vi "Logo Exaprom.vi"(0 "PDFStamper GetOverContent":refnum<k24>, 1 "text1":string="Exaprom inc.", 3 "Text2":string="Consultation et essais en génie des\nmatériaux et en énergies durables", 9 "Facteur":sgl=0.2, 11 "error in (no error)":errorcluster, 13 "Page dimensions":T1={"Start at page"=1, "Orientation"=enum."Portrait", "widht"=612.0, "height"=792.0, "Margin left"=72.0, "Margin right"=72.0, "Margin top"=72.0, "Margin bottom"=72.0}) -> (4 "PDFStamper GetOverContent duplicate":refnum<k24>, 15 "error out":errorcluster)   [LabVIEW 2013]
doc: "Version 1.0\nDeveloped by Jean-Marc Simard\nCopyright © 2010, Exaprom Inc.\nAll rights reserved.\nLicense: BSD\n\nWith iTextSharp Library\n(http://itextsharp.sourceforge.net)"
uses:
  C:/Users/MaxCorp/Documents/GitHub/TopView/DLL/itextsharp.dll
  DLL/itextsharp.dll
  Controls/Header footer horiz alignment.ctl
  Controls/Font size.ctl
  Controls/Font color.ctl
  Controls/Font cluster.ctl
  Controls/Cell Vertical alignment.ctl
  Controls/Page Orientation.ctl
  Controls/Page dimensions.ctl
panel:
  in  "Alignment":T3
  in  "Vertical Alignement":T4=enum."BOTTOM"
  # "Consultation et essais en génie des\nmatériaux et en énergies durables"
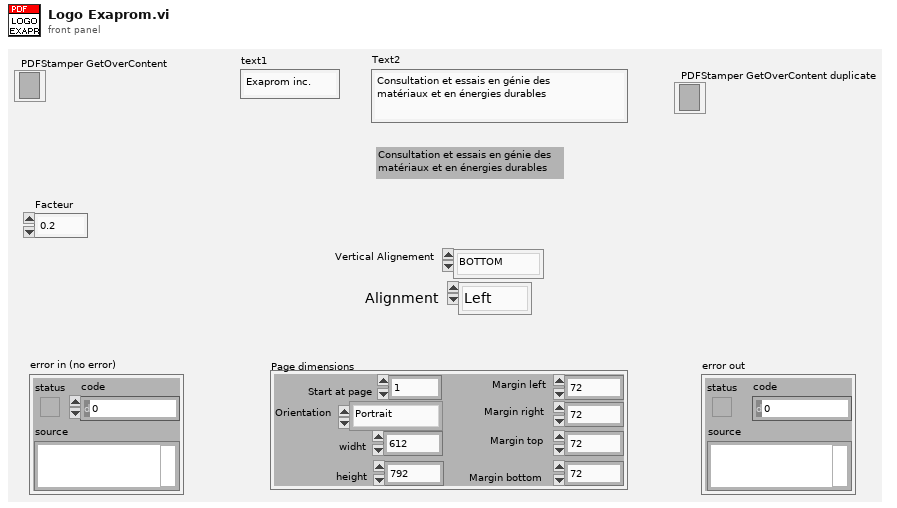
[diagram p1: front panel]
types:
  T1 = typedef "Page dimensions.ctl" = cluster{"Start at page":i32, "Orientation":T2, "widht":sgl, "height":sgl, "Margin left":sgl, "Margin right":sgl, "Margin top":sgl, "Margin bottom":sgl}
  T2 = typedef "Page Orientation.ctl" = enum16{"Portrait", "Landscape"}
  T3 = typedef "Header footer horiz alignment.ctl" = enum16{"Left", "Center", "Right"}
  T4 = typedef "Cell Vertical alignment.ctl" = enum16{"TOP", "MIDDLE", "BOTTOM"}
  T5 = typedef "Font size.ctl" = sgl
  T6 = typedef "Font cluster.ctl" = cluster{"Name":string, "Size":T5, "Color":T7, "Style":cluster{"Bold":bool, "Italic":bool, "Underline":bool, "Strikeout":bool}}
  T7 = typedef "Font color.ctl" = u32
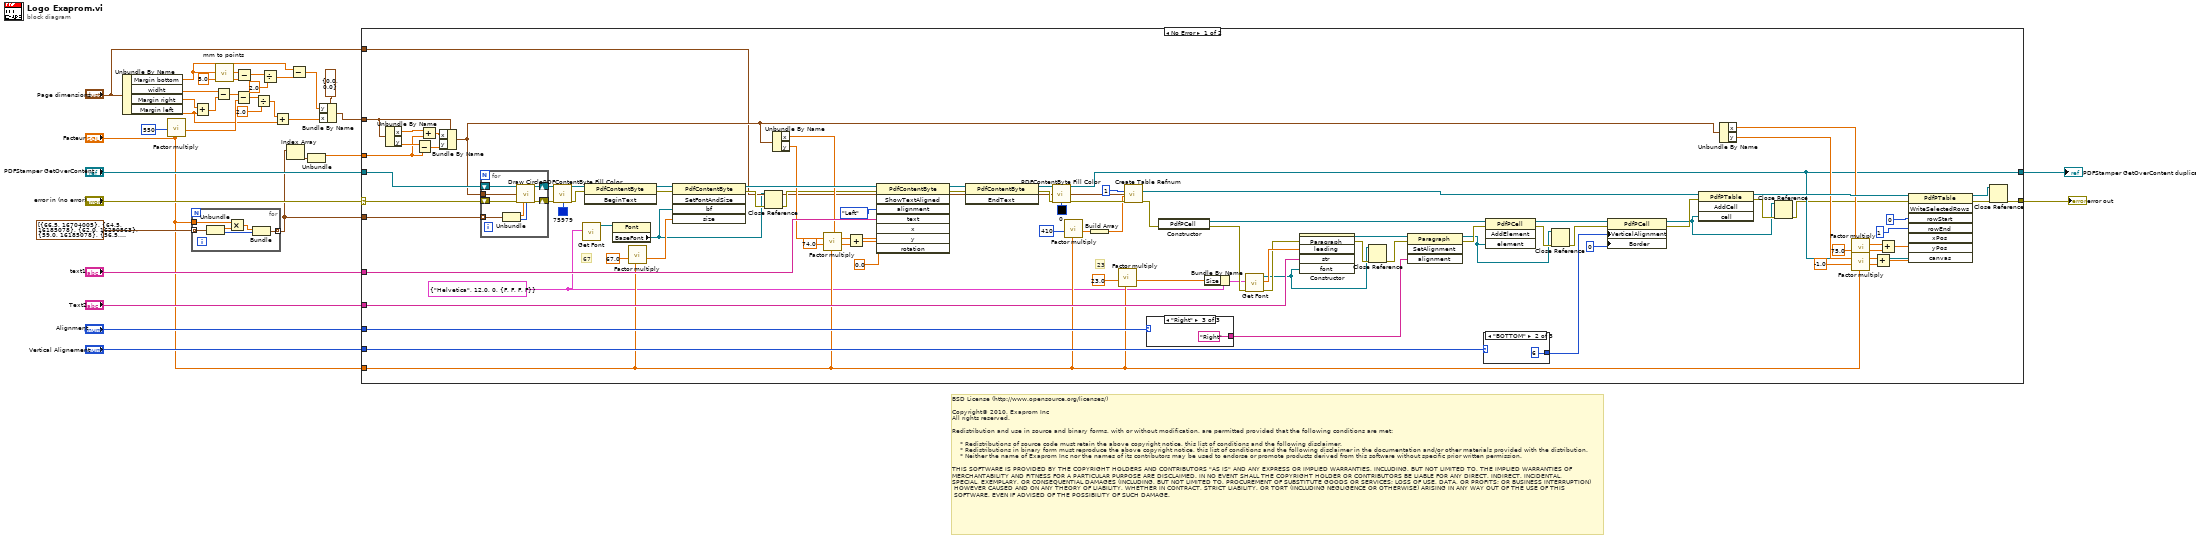
[diagram p0: block diagram]
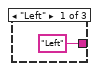
[diagram p2: hidden frame]
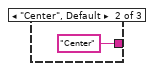
[diagram p3: hidden frame]
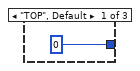
[diagram p4: hidden frame]
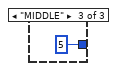
[diagram p5: hidden frame]
diagram:
  # "BSD License (http://www.opensource.org/licenses/)\n\nCopyright© 2010, Exaprom Inc\nAll rights reserved.\n\nRedistribution and use in source and binary forms, with or without modification, are permitted provided that the following conditions are met:\n\n    * Redistributions of source code must retain the above copyright notice, this list of conditions and the following disclaimer.\n    * Redistributions in binary form must reproduce the above copyright notice, this list of conditions and the following disclaimer in the documentation and/or other materials provided with the distribution.\n    * Neither the name of Exaprom Inc nor the names of its contributors may be used to endorse or promote products derived from this software without specific prior written permission.\n\nTHIS SOFTWARE IS PROVIDED BY THE COPYRIGHT HOLDERS AND CONTRIBUTORS \"AS IS\" AND ANY EXPRESS OR IMPLIED WARRANTIES, INCLUDING, BUT NOT LIMITED TO, THE IMPLIED WARRANTIES OF \nMERCHANTABILITY AND FITNESS FOR A PARTICULAR PURPOSE ARE DISCLAIMED. IN NO EVENT SHALL THE COPYRIGHT HOLDER OR CONTRIBUTORS BE LIABLE FOR ANY DIRECT, INDIRECT, INCIDENTAL,\nSPECIAL, EXEMPLARY, OR CONSEQUENTIAL DAMAGES (INCLUDING, BUT NOT LIMITED TO, PROCUREMENT OF SUBSTITUTE GOODS OR SERVICES; LOSS OF USE, DATA, OR PROFITS; OR BUSINESS INTERRUPTION)\n HOWEVER CAUSED AND ON ANY THEORY OF LIABILITY, WHETHER IN CONTRACT, STRICT LIABILITY, OR TORT (INCLUDING NEGLIGENCE OR OTHERWISE) ARISING IN ANY WAY OUT OF THE USE OF THIS\n SOFTWARE, EVEN IF ADVISED OF THE POSSIBILITY OF SUCH DAMAGE."
  n1 = Unbundle By Name("Page dimensions") -> ("Margin bottom"=w4:sgl, "widht"=w27:sgl, "Margin right"=w26:sgl, "Margin left"=w20:sgl)
  n2 = call "Factor multiply.vi"("factor"="Facteur", "Numeric IN"=550) -> ("Numeric OUT"=w23:sgl)  [unwired: 6 out]
  n3 = for {
    tunnel: cluster{"r":sgl, "Color":u32}[] [{"r"=66.5, "Color"=16704005}, {"r"=64.5, "Color"=16185078}, {"r"=62.0, "Color"=16290563}, {"r"=59.0, "Color"=16185078}, {"r"=56.5, "Color"=16290563}, {"r"=52.5, "Color"=16185078}, {"r"=50.0, "Color"=16711680}] -> [w40] mode=indexing
    tunnel: "Facteur" -> [w38]
    tunnel: [w35] -> w12 mode=indexing
    n4 = Unbundle(w40) -> ("r"=w39:sgl, "Color"=w36:u32)
    n5 = Multiply(x=w38, y=w39) -> (x*y=w37:sgl)
    n6 = Bundle(w37, "Color"=w36) -> (w35:cluster{sgl, "Color":u32})  [unwired: 1 out]
  }
  n7 = Add(x=w26, y=w20) -> (x+y=w25:sgl)
  n8 = Subtract(x=w27, y=w25) -> (x-y=w24:sgl)
  n9 = call "mm to points.vi"("mm"=sgl 5.0) -> ("points"=w10:sgl)  [unwired: 4 out]
  n10 = Subtract(x=w24, y=w23) -> (x-y=w22:sgl)
  n11 = Subtract(x=w4, y=w10) -> (x-y=w6:sgl)
  n12 = Divide(x=w22, y=2.0) -> (x/y=w8:dbl)
  n13 = Divide(x=w6, y=2.0) -> (x/y=w5:dbl)
  n14 = Add(x=w8, y=w20) -> (x+y=w19:dbl)
  n15 = Index Array(array=w12) -> (element=w13:cluster{sgl, "Color":u32})  [unwired: 1 in]
  n16 = Subtract(x=w4, y=w5) -> (x-y=w2:dbl)
  n17 = Unbundle(w13) -> (w11:sgl)  [unwired: 1 out]
  n18 = Bundle By Name(cluster=cluster{"x":sgl, "y":sgl} {"x"=0.0, "y"=0.0} ("Position"), "y"=w2, "x"=w19) -> (w18:cluster{"x":sgl, "y":sgl})
  n19 = case shown="No Error" "error in (no error)" {
    selector: "error in (no error)" -> [w61 w144]
    tunnel: [w96 w144] -> w33
    tunnel: w18 -> [w67 _]
    tunnel: "Facteur" -> [w60 _]
    tunnel: "text1" -> [w92 _]
    tunnel: "Text2" -> [w88 _]
    tunnel: "Alignment" -> [w87 _]
    tunnel: "Vertical Alignement" -> [w86 _]
    tunnel: "PDFStamper GetOverContent" -> [w62 w143]
    tunnel: [w65 w143] -> w16
    tunnel: w12 -> [w58 _]
    tunnel: w11 -> [w57 _]
    tunnel: "Page dimensions" -> [w44 _]
    frame No Error {
      w42 = T6 {"Name"="Helvetica", "Size"=12.0, "Color"=0, "Style"={"Bold"=FALSE, "Italic"=FALSE, "Underline"=FALSE, "Strikeout"=FALSE}} ("Font")
      # "23"
      # "67"
      n20 = Unbundle By Name(w67) -> ("x"=w71:sgl, "y"=w70:sgl)
      n21 = Subtract(x=w70, y=w57) -> (x-y=w68:sgl)
      n22 = Add(x=w71, y=w57) -> (x+y=w69:sgl)
      n23 = Bundle By Name(cluster=w67, "x"=w69, "y"=w68) -> (w59:cluster{"x":sgl, "y":sgl})
      n24 = for {
        tunnel: w58 -> [w136] mode=indexing
        shift-right: [w133] -> w64
        shift-left: w62 -> [w134]
        shift-right: [w132] -> w63
        shift-left: w61 -> [w131]
        tunnel: w59 -> [w130]
        n25 = Unbundle(w136) -> (w129:sgl, "Color"=w135:u32)
        n26 = call "Draw Circle.vi"("GetOverContent IN"=w134, "Center"=w130, "error in (no error)"=w131, "r"=w129, "Color Box"=w135) -> ("GetOverContent OUT"=w133:refnum<k24>, "error out"=w132:errorcluster)  [unwired: 1 in, 8 out]
      }
      n27 = call "PDFContentByte Fill Color.vi"("PDFContentByte"=w64, "error in (no error)"=w63, "Color Box"=u32 75979) -> ("PDFContentByte duplicate"=w45:refnum<k24>, "error out"=w124:errorcluster)  [unwired: 1 in, 10 out]
      n28 = call "Get Font.vi"("Font IN"=w42) -> ("Font"=w43:refnum<k24>)  [unwired: 7 in, 3 out]
      n29 = invoke class="PdfContentByte" method="BeginText"(reference=w45, error in=w124) -> (reference out=w117:refnum<k24>, error out=w122:errorcluster)  [unwired: 1 in, 1 out]
      n30 = property class="Font"(reference=w43) -> ("BaseFont"=w41:refnum<k24>)  [unwired: 1 in, 2 out]
      n31 = call "Factor multiply.vi"("factor"=w60, "Numeric IN"=sgl 67.0 ("size")) -> ("Numeric OUT"=w115:sgl)  [unwired: 6 out]
      n32 = invoke class="PdfContentByte" method="SetFontAndSize"(reference=w117, error in=w122, "bf"=w41, "size"=w115) -> (reference out=w121:refnum<k24>, error out=w56:errorcluster)  [unwired: 1 in, 3 out]
      n33 = Close Reference(reference=w41, error in (no error)=w56) -> (error out=w55:errorcluster)
      n34 = Unbundle By Name(w59) -> ("x"=w84:sgl, "y"=w85:sgl)
      n35 = call "Factor multiply.vi"("factor"=w60, "Numeric IN"=sgl 74.0 ("y")) -> ("Numeric OUT"=w82:sgl)  [unwired: 6 out]
      n36 = Add(x=w84, y=w82) -> (x+y=w81:sgl)
      n37 = invoke class="PdfContentByte" method="ShowTextAligned"(reference=w121, error in=w55, "alignment"=Header_footer_horiz_alignment."Left" ("Alignment 2"), "text"=w92, "x"=w81, "y"=w85, "rotation"=sgl 0.0) -> (reference out=w119:refnum<k24>, error out=w123:errorcluster)  [unwired: 1 in, 6 out]
      n38 = invoke class="PdfContentByte" method="EndText"(reference=w119, error in=w123) -> (reference out=w126:refnum<k24>, error out=w127:errorcluster)  [unwired: 1 in, 1 out]
      n39 = call "PDFContentByte Fill Color.vi"("PDFContentByte"=w126, "error in (no error)"=w127, "Color Box"=u32 0) -> ("PDFContentByte duplicate"=w65:refnum<k24>, "error out"=w97:errorcluster)  [unwired: 1 in, 10 out]
      n40 = call "Factor multiply.vi"("factor"=w60, "Numeric IN"=410) -> ("Numeric OUT"=w94:sgl)  [unwired: 6 out]
      n41 = Build Array(w94) -> (w93:sgl[])
      n42 = call "Factor multiply.vi"("factor"=w60, "Numeric IN"=T5 23.0 ("Size")) -> ("Numeric OUT"=w90:sgl)  [unwired: 6 out]
      n43 = call "Create Table Refnum.vi"("columnWidth (points)"=w93, "Table properties"=w44, "error in (no error)"=w97, "numColumns"=1) -> ("error out"=w111:errorcluster, "PdfP Table ref"=w112:refnum<k24>)  [unwired: 3 in, 1 out]
      n44 = case shown="\"Right\"" w87 {
        tunnel: ["Left" "Center" "Right"] -> w105
        frame "Left" {
        }
        frame "Center", Default {
        }
        frame "Right" {
        }
      }
      n45 = constructor class="PdfPCell"(error in=w111) -> (reference out=w106:refnum<k24>, error out=w107:errorcluster)  [unwired: 2 in, 1 out]
      n46 = Bundle By Name(cluster=w42, "Size"=w90) -> (w89:T6)
      n47 = call "Get Font.vi"("error in (no error)"=w107, "Font IN"=w89) -> ("error out"=w108:errorcluster, "Font Size"=w110:T5, "Font"=w52:refnum<k24>)  [unwired: 1 in, 6 out]
      n48 = constructor class="Paragraph"(error in=w108, "leading"=w110, "str"=w88, "font"=w52) -> (reference out=w104:refnum<k24>, error out=w54:errorcluster)  [unwired: 2 in, 4 out]
      n49 = Close Reference(reference=w52, error in (no error)=w54) -> (error out=w53:errorcluster)
      n50 = invoke class="Paragraph" method="SetAlignment"(reference=w104, error in=w53, "alignment"=w105) -> (reference out=w50:refnum<k24>, error out=w66:errorcluster)  [unwired: 1 in, 2 out]
      n51 = case shown="\"BOTTOM\"" w86 {
        tunnel: [0 6 5] -> w103
        frame "TOP", Default {
        }
        frame "BOTTOM" {
        }
        frame "MIDDLE" {
        }
      }
      n52 = invoke class="PdfPCell" method="AddElement"(reference=w106, error in=w66, "element"=w50) -> (reference out=w102:refnum<k24>, error out=w51:errorcluster)  [unwired: 1 in, 2 out]
      n53 = Close Reference(reference=w50, error in (no error)=w51) -> (error out=w49:errorcluster)
      n54 = property class="PdfPCell"(reference=w102, error in=w49, "VerticalAlignment"=w103, "Border"=0) -> (reference out=w47:refnum<k24>, error out=w109:errorcluster)
      n55 = invoke class="PdfPTable" method="AddCell"(reference=w112, error in=w109, "cell"=w47) -> (reference out=w113:refnum<k24>, error out=w48:errorcluster)  [unwired: 1 in, 2 out]
      n56 = Unbundle By Name(w59) -> ("x"=w73:sgl, "y"=w77:sgl)
      n57 = Close Reference(reference=w47, error in (no error)=w48) -> (error out=w46:errorcluster)
      n58 = call "Factor multiply.vi"("factor"=w60, "Numeric IN"=sgl 75.0 ("y")) -> ("Numeric OUT"=w75:sgl)  [unwired: 6 out]
      n59 = call "Factor multiply.vi"("factor"=w60, "Numeric IN"=sgl -1.0 ("y")) -> ("Numeric OUT"=w80:sgl)  [unwired: 6 out]
      n60 = Add(x=w77, y=w80) -> (x+y=w76:sgl)
      n61 = Add(x=w73, y=w75) -> (x+y=w72:sgl)
      n62 = invoke class="PdfPTable" method="WriteSelectedRows"(reference=w113, error in=w46, "rowStart"=0, "rowEnd"=1, "xPos"=w72, "yPos"=w76, "canvas"=w65) -> (reference out=w101:refnum<k24>, error out=w100:errorcluster)  [unwired: 1 in, 6 out]
      n63 = Close Reference(reference=w101, error in (no error)=w100) -> (error out=w96:errorcluster)
    }
    frame Error {
    }
  }
  "error out" <- w33
  "PDFStamper GetOverContent duplicate" <- w16
